vi "dfd_FXP Symmetric FIR with IS.vi"(6 "state in":i64[](array[numeric]), 7 "FXPOPs":T5[](array[typedef]) {"source" items=["Coef a/k"=0, "Coef b/v"=7, "Input"=1, "Output"=2, "Multiplicand"=3, "Product"=4, "Sum"=5, "Delay"=6, "Gain"=8]}, 8 "filtering statistics in":T4(array[cluster]) {"statistics information"."min value" format="%.2f"; "statistics information"."max value" format="%.2f"; "Quantizer Source" items=["Coefficients a/k"=0, "Coefficients b/v"=7, "Input"=1, "Output"=2, "Multiplicand"=3, "Product"=4, "Sum"=5, "Delay"=6]}, 10 "coef b":T7, 11 "X":T7) -> (0 "filtering statistics out":T4(array[cluster]) {"statistics information"."min value" format="%.2f"; "statistics information"."max value" format="%.2f"; "Quantizer Source" items=["Coefficients a/k"=0, "Coefficients b/v"=7, "Input"=1, "Output"=2, "Multiplicand"=3, "Product"=4, "Sum"=5, "Delay"=6]}, 3 "filtered X":T7, 4 "state out":i64[](array[numeric]))   [LabVIEW 2017, in "NI_DigFilter_FXP.lvlib"]
uses:
  <vilib>/addons/Digital Filter Design/NI_DigFilter_FXP.lvlib
  <vilib>/addons/Digital Filter Design/_Objects.llb/dfd_DFXP Data Type (vector).ctl
  <vilib>/addons/Digital Filter Design/_Objects.llb/dfd_DFXP Operation Parameter.ctl
  <vilib>/addons/Digital Filter Design/_Objects.llb/dfd_Internal Quantization Srcs.ctl
  <vilib>/addons/Digital Filter Design/_Objects.llb/DFD Quantization Sources.ctl
  <vilib>/addons/Digital Filter Design/_Objects.llb/DFD FXP Statistics Data.ctl
  <vilib>/addons/Digital Filter Design/_Objects.llb/dfd_DFXP Data Type (scaler).ctl
  <vilib>/addons/Digital Filter Design/NI_DigFilterLicensed.lvlib
panel:
  in  "DFXP Value":T1={"value"=0, "wl"=0, "iwl"=0, "Signed"=TRUE} {"value" format="%.0x"}
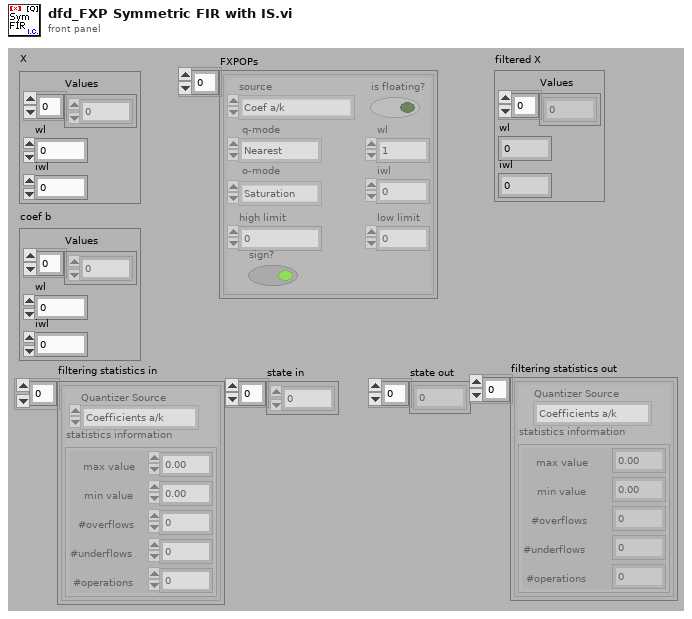
[diagram p1: front panel]
types:
  T1 = typedef "dfd_DFXP Data Type (scaler).ctl" = cluster{"value":i64, "wl":i16, "iwl":i16, "Signed":bool}
  T2 = typedef "NI_DigFilterLicensed.lvlib/DFD Quantization Sources.ctl" = u16
  T3 = typedef "NI_DigFilterLicensed.lvlib/DFD FXP Statistics Data.ctl" = cluster{"max value":ext, "min value":ext, "#overflows":i32, "#underflows":i32, "#operations":i32}
  T4 = cluster{"Quantizer Source":T2, "statistics information":T3}[]
  T5 = typedef "dfd_DFXP Operation Parameter.ctl" = cluster{"source":T6, "is floating?":bool, "o-mode":enum16{"Saturation", "Wrap"}, "q-mode":enum16{"Nearest", "Truncation"}, "wl":i16, "high limit":i64, "low limit":i64, "iwl":i16, "sign?":bool}
  T6 = typedef "NI_DigFilterLicensed.lvlib/dfd_Internal Quantization Srcs.ctl" = u16
  T7 = typedef "dfd_DFXP Data Type (vector).ctl" = cluster{"Values":i64[], "wl":i16, "iwl":i16}
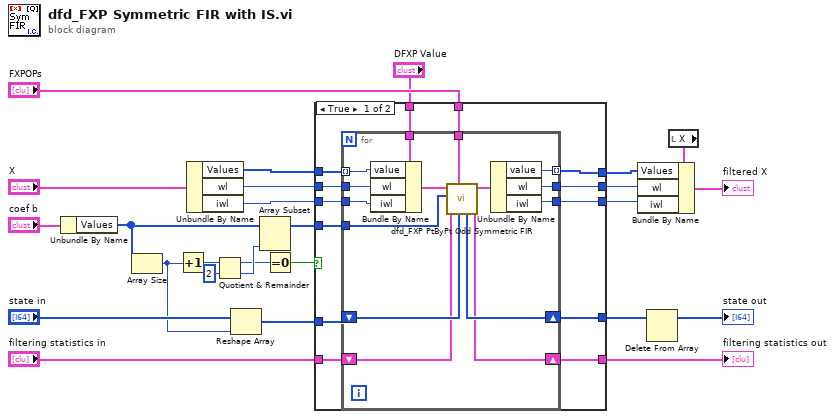
[diagram p0: block diagram]
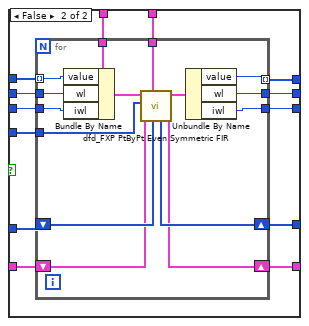
[diagram p2: hidden frame]
diagram:
  n1 = Unbundle By Name("coef b") -> ("Values"=w10:i64[])
  n2 = Array Size(array=w10) -> (size(s)=w18:i32)
  n3 = Increment(x=w18) -> (x+1=w24:i32)
  n4 = Unbundle By Name("X") -> ("Values"=w9:i64[], "wl"=w7:i16, "iwl"=w6:i16)
  n5 = Quotient & Remainder(x=w24, y=2) -> (x-y*floor(x/y)=w17:i32, floor(x/y)=w22:i32)
  n6 = Reshape Array("state in", w18) -> (w19:i64[])
  n7 = Array Subset(array=w10, length=w22) -> (w23:i64[])  [unwired: 1 in]
  n8 = Equal To 0?(x=w17) -> (x = 0?=w13:bool)
  n9 = case shown="True" w13 {
    tunnel: [w39 w67] -> w16
    tunnel: w9 -> [w38 w66]
    tunnel: w23 -> [w37 w65]
    tunnel: w19 -> [w36 w64]
    tunnel: [w35 w63] -> w5
    tunnel: "FXPOPs" -> [w34 w62]
    tunnel: "filtering statistics in" -> [w33 w61]
    tunnel: [w32 w60] -> w11
    tunnel: "DFXP Value" -> [w31 w59]
    tunnel: w7 -> [w30 w58]
    tunnel: w6 -> [w29 w57]
    tunnel: [w28 w56] -> w2
    tunnel: [w27 w55] -> w1
    frame True {
      n10 = for {
        tunnel: w38 -> [w53] mode=indexing
        tunnel: w37 -> [w49]
        shift-right: [w50] -> w39
        shift-left: w36 -> [w51]
        tunnel: [w42] -> w35 mode=indexing
        tunnel: w34 -> [w54]
        shift-right: [w47] -> w32
        shift-left: w33 -> [w48]
        tunnel: w31 -> [w45]
        tunnel: w30 -> [w44]
        tunnel: w29 -> [w43]
        tunnel: [w41] -> w28
        tunnel: [w40] -> w27
        n11 = Bundle By Name(cluster=w45, "value"=w53, "wl"=w44, "iwl"=w43) -> (w46:T1)
        n12 = call <vilib>:"dfd_FXP PtByPt Odd Symmetric FIR.vi"("state in"=w51, "FXPOPs"=w54, "filtering statistics in"=w48, "coef b (half stored)"=w49, "x"=w46) -> ("filtering statistics out"=w47:T4, "filtered x"=w52:T1, "state out"=w50:i64[])  [unwired: 4 out]
        n13 = Unbundle By Name(w52) -> ("value"=w42:i64, "wl"=w41:i16, "iwl"=w40:i16)
      }
    }
    frame False {
      n14 = for {
        tunnel: w66 -> [w75] mode=indexing
        tunnel: w65 -> [w81]
        shift-right: [w79] -> w67
        shift-left: w64 -> [w80]
        tunnel: [w70] -> w63 mode=indexing
        tunnel: w62 -> [w82]
        shift-right: [w77] -> w60
        shift-left: w61 -> [w78]
        tunnel: w59 -> [w76]
        tunnel: w58 -> [w74]
        tunnel: w57 -> [w73]
        tunnel: [w69] -> w56
        tunnel: [w68] -> w55
        n15 = Bundle By Name(cluster=w76, "value"=w75, "wl"=w74, "iwl"=w73) -> (w72:T1)
        n16 = call <vilib>:"dfd_FXP PtByPt Even Symmetric FIR.vi"("state in"=w80, "FXPOPs"=w82, "filtering statistics in"=w78, "coef b (half stored)"=w81, "x"=w72) -> ("filtering statistics out"=w77:T4, "filtered x"=w71:T1, "state out"=w79:i64[])  [unwired: 4 out]
        n17 = Unbundle By Name(w71) -> ("value"=w70:i64, "wl"=w69:i16, "iwl"=w68:i16)
      }
    }
  }
  "filtering statistics out" <- w11
  n18 = Delete From Array(array=w16) -> (array with subset deleted=→"state out":i64[])  [unwired: 2 in, 1 out]
  n19 = local read "X"() -> (w4:T7)
  n20 = Bundle By Name(cluster=w4, "Values"=w5, "wl"=w2, "iwl"=w1) -> (→"filtered X":T7)
